vi "YAML.AddSections.vi"(2 "Section 2":string, 3 "Section 1":string) -> (1 "Output":string)   [LabVIEW 2016, in "AFM Control.lvclass"]
uses:
  AFM Control.lvclass
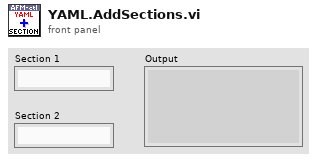
[diagram p1: front panel]
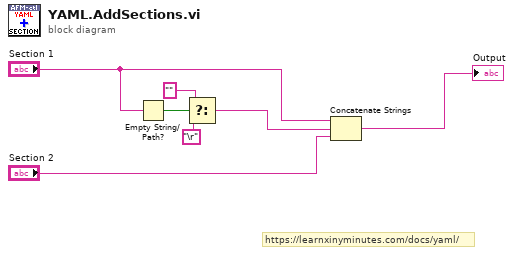
[diagram p0: block diagram]
diagram:
  # "https://learnxinyminutes.com/docs/yaml/"
  n1 = Empty String/Path?(string/path="Section 1") -> (empty?=w5:bool)
  n2 = Select(t="", s=w5, f="\r") -> (s? t:f=w2:string)
  n3 = Concatenate Strings("Section 1", w2, "Section 2") -> (→"Output":string)
